vi "create_connection.vi"(0 "device_index (def=0)":i32, 11 "error in (no error)":errorcluster, 12 "clear_buffer? (T)":bool=TRUE) -> (4 "reference":i32, 15 "error out":errorcluster)   [LabVIEW 2012]
doc: "Opens a reference to the specified device (takes as input device Index and outputs a device Reference). \n\nImplementss the USB Communication API function \"fnPerformaxCaomOpen\".\n\nNOTE: The \"index\" is determined by choosing the item from a list of queried items using the \"get_device_list.vi\" VI. Further note a USB Clear Buffer command is (by default) issued immediately after a connection is established in the event a previous session was not properly terminated. This feature is NOT supported in all versions of the API - therefore it may be bypassed by assigning a FALSE to the \"clear_buffer\" input.\n\nProduced By:\n\nChristopher Lemieux\nKod Integrations, LLC\n4835 Marianne Drive\nMount Airy, MD 21771\nhttp://www.kodintegrations.com\nemail: clemieux@kodintegrations.com\nphone: (240) 687-1288"
uses:
  support/controls/errors_actions.ctl
  PerformaxCom.dll
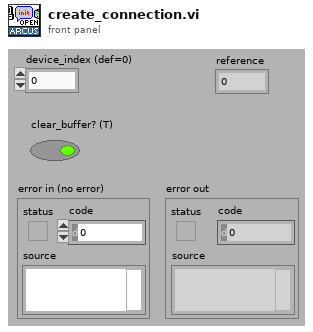
[diagram p1: front panel]
types:
  T1 = typedef "errors_actions.ctl" = enum16{"clearBuff", "closeRef", "noDeviceInfo", "noDevices", "openRef", "sendReceive", "setTimeouts", "unknown"}
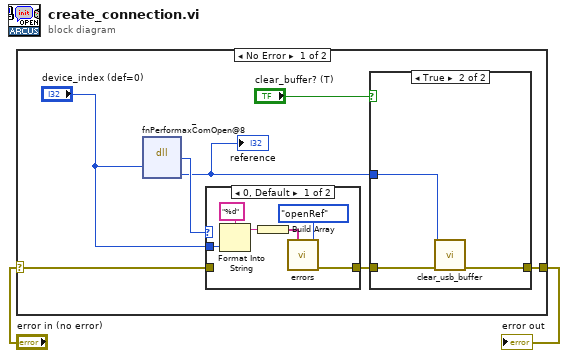
[diagram p0: block diagram]
diagram:
  n1 = case shown="No Error" "error in (no error)" {
    selector: "error in (no error)" -> [w7 w21]
    tunnel: [w4 w21] -> w1
    frame No Error {
      n2 = dll-call lib="PerformaxCom.dll" fn="_fnPerformaxComOpen@8"("deviceIndex"="device_index (def=0)") -> ("success"=w9:i32, "reference"=w3:i32)  [unwired: 5 in, 2 out]
      "reference" <- w3
      n3 = case shown="0, Default" w9 {
        tunnel: [w18 w20] -> w5
        tunnel: w7 -> [_ w20]
        tunnel: "device_index (def=0)" -> [w17 _]
        frame 0, Default {
          n4 = Format Into String(format string="%d", w17) -> (resulting string=w15:string)  [unwired: 2 in, 1 out]
          n5 = Build Array(w15) -> (w14:string[])
          n6 = call "errors.vi"("errors"=errors_actions."openRef", "supp_text"=w14) -> ("error out"=w18:errorcluster)  [unwired: 13 in]
        }
        frame 1 {
        }
      }
      n7 = case shown="True" "clear_buffer? (T)" {
        tunnel: w5 -> [w10 w13]
        tunnel: [w10 w12] -> w4
        tunnel: w3 -> [_ w11]
        frame False {
        }
        frame True {
          n8 = call "clear_usb_buffer.vi"("reference"=w11, "error in (no error)"=w13) -> ("error out"=w12:errorcluster)  [unwired: 17 in]
        }
      }
    }
    frame Error {
    }
  }
  "error out" <- w1
